vi "Compare timing results.vi"() -> ()   [LabVIEW 2009]
uses:
  <vilib>/Utility/file.llb/Read From Spreadsheet File (DBL).vi
panel:
  out "XY Graph":cluster{"all rows":dbl[], "all rows":dbl[]}[](graph)
  in  "stop":bool
  out "element":string
  in  "index":i32
  in  "Load":bool
  out "Available files":string[](array[string])
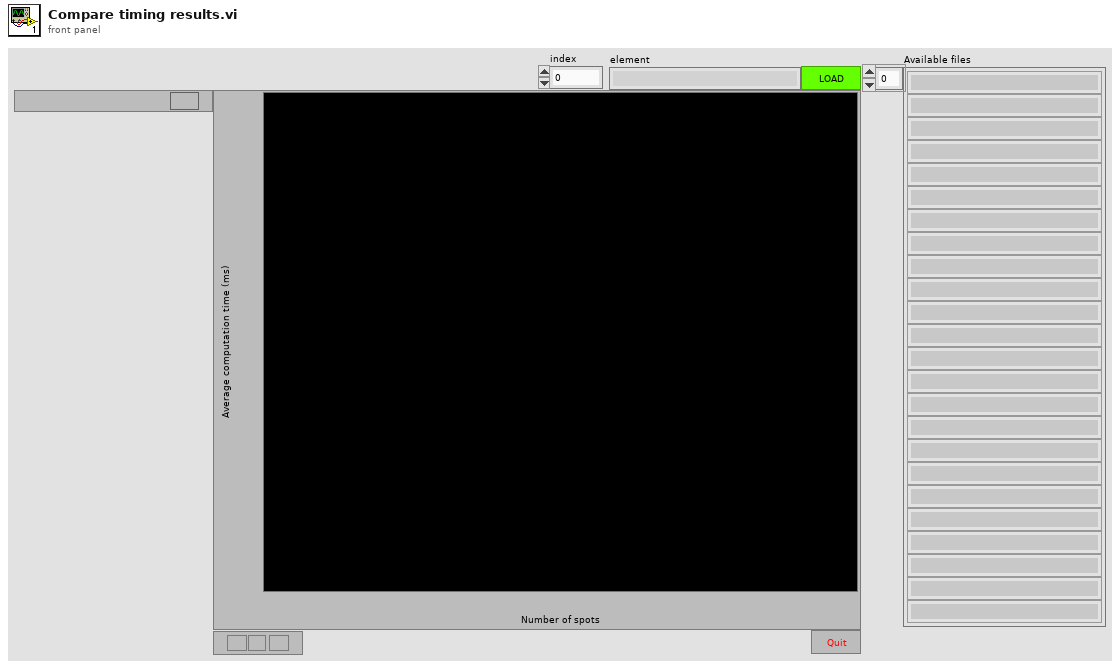
[diagram p1: front panel]
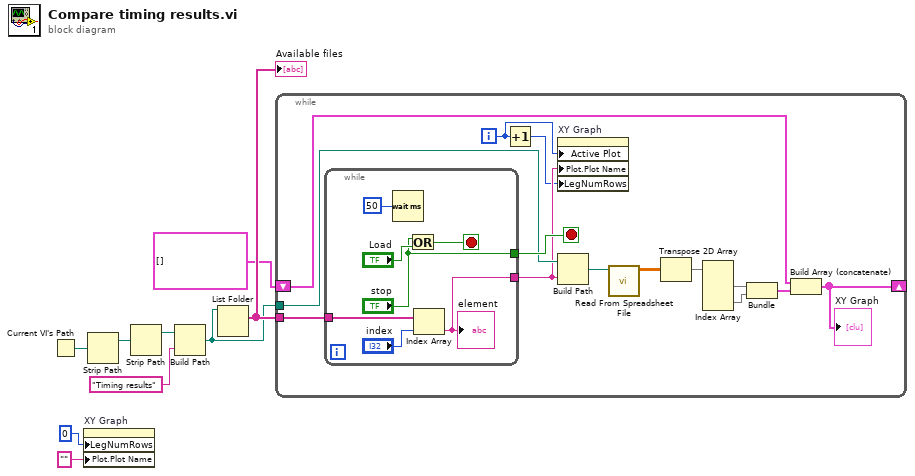
[diagram p0: block diagram]
diagram:
  n1 = Current VI's Path() -> (path=w8:path)
  n2 = property on="XY Graph" class="XYGraph (strict)"("LegNumRows"=u32 0 ("Legend:Number of Rows"), "Plot.Plot Name"="") -> ()  [unwired: 2 in, 2 out]
  n3 = Strip Path(path=w8) -> (stripped path=w3:path)  [unwired: 1 out]
  n4 = Strip Path(path=w3) -> (stripped path=w7:path)  [unwired: 1 out]
  n5 = Build Path(base path=w7, name or relative path="Timing results") -> (appended path=w5:path)
  n6 = List Folder(path=w5) -> (filenames=w6:string[])  [unwired: 3 in, 3 out]
  "Available files" <- w6
  n7 = while {
    tunnel: w6 -> [w23]
    tunnel: w5 -> [w17]
    shift-right: [w14] -> _
    shift-left: cluster{dbl[], dbl[]}[] [] -> [w13]
    i -> [w11]
    stop <- w18 stop-if-true
    n8 = while {
      tunnel: w23 -> [w27]
      tunnel: [w26] -> w12
      tunnel: ["stop"] -> w18
      stop <- w25 stop-if-true
      n9 = Wait (ms)(milliseconds to wait=u32 50) -> ()  [unwired: 1 out]
      n10 = Or(x="stop", y="Load") -> (x .or. y?=w25:bool)
      n11 = Index Array(array=w27, index="index") -> (element=w26:string)
      "element" <- w26
    }
    n12 = Increment(x=w11) -> (x+1=w10:i32)
    n13 = property on="XY Graph" class="XYGraph (strict)"("Active Plot"=w11, "Plot.Plot Name"=w12, "LegNumRows"=w10) -> ()  [unwired: 2 in, 2 out]
    n14 = Build Path(base path=w17, name or relative path=w12) -> (appended path=w16:path)
    n15 = call-poly <vilib>:"Read From Spreadsheet File.vi"("file path (dialog if empty)"=w16) -> ("all rows"=w22:dbl[][])  [unwired: 6 in, 4 out]
    n16 = Transpose 2D Array(2D array=w22) -> (transposed array=w15:dbl[][])
    n17 = Index Array(array=w15) -> (element #1=w21:dbl[], element #2=w20:dbl[])  [unwired: 4 in]
    n18 = Bundle(w21, w20) -> (w19:cluster{dbl[], dbl[]})  [unwired: 1 in]
    n19 = Build Array (concatenate)(w13, w19) -> (w14:cluster{dbl[], dbl[]}[])
    "XY Graph" <- w14
  }
